vi "waitOnProcessExit.vi"(6 "Timeout Exit":i32, 8 "error in (no error)":errorcluster {"code" format="Error %.0f"}, 9 "Message":string, 10 "MHL":refnum<queue>, 11 "notifier":refnum<notifier>) -> (0 "error out":errorcluster {"code" format="Error %.0f"}, 2 "MHLDup":refnum<queue>, 3 "processExit?":bool)   [LabVIEW 2017]
doc: "This VI checks for exitProcess notificaiton from a subpanel process. If received, processExit = True. Otherwise the input waitOnProcess message will be enqued to the MHLQueue."
uses:
  Message Queues/Message Cluster.ctl
  Message Queues/Message Queue.lvlib
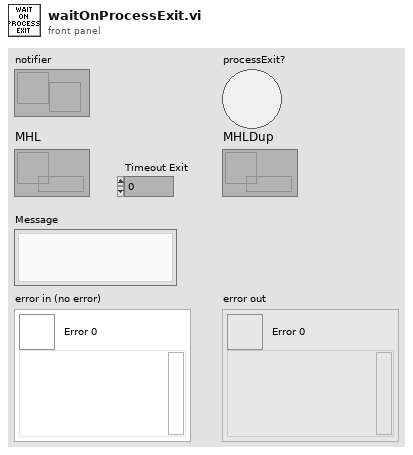
[diagram p1: front panel]
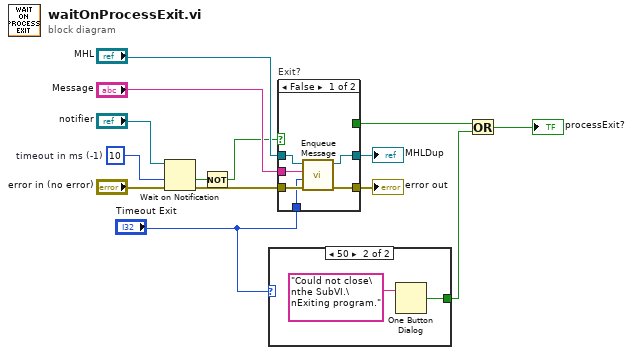
[diagram p0: block diagram]
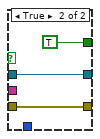
[diagram p3: hidden frame]
diagram:
  w10 = 10  # timeout in ms (-1)
  n1 = Wait on Notification(notifier="notifier", timeout in ms (-1)=w10, error in (no error)="error in (no error)") -> (timed out?=w6:bool, error out=w12:errorcluster)  [unwired: 1 in, 2 out]
  n2 = Not(x=w6) -> (.not. x?=w4:bool)
  n3 = case shown="50" "Timeout Exit" {
    tunnel: [_ w15] -> w1
    frame 0, Default {
    }
    frame 50 {
      n4 = One Button Dialog(message="Could not close\nthe SubVI.\nExiting program.") -> (true=w15:bool)  [unwired: 1 in]
    }
  }
  n5 = case "Exit?" shown="False" w4 {
    tunnel: w12 -> [w22 w25]
    tunnel: [w21 w25] -> w13
    tunnel: [w18 w23] -> w7
    tunnel: [_ TRUE] -> w3
    tunnel: "MHL" -> [w20 w23]
    tunnel: "Message" -> [w19 _]
    tunnel: "Timeout Exit" -> [w17 _]
    frame False {
      n6 = call "Enqueue Message.vi"("error in (no error)"=w22, "Message Data"=w17, "Message"=w19, "Message Queue"=w20) -> ("error out"=w21:errorcluster, "dup Message Queue"=w18:refnum<queue>)  [unwired: 6 in]
    }
    frame True {
    }
  }
  "error out" <- w13
  "MHLDup" <- w7
  n7 = Or(x=w3, y=w1) -> (x .or. y?=→"processExit?":bool)
